vi "get_message.vi"(8 "error in (no error)":errorcluster, 11 "MoAgSy_Message.lvclass in":refnum<class "MoAgSy_Message.lvclass">) -> (0 "error out":errorcluster, 2 "Message":string, 3 "MoAgSy_Message.lvclass out":refnum<class "MoAgSy_Message.lvclass">)   [LabVIEW 2009, in "MoAgSy.lvlib" / "MoAgSy_Message.lvclass"]
uses:
  MoAgSy_Message.lvclass
  MoAgSy_Message.lvclass/MoAgSy_Message.ctl
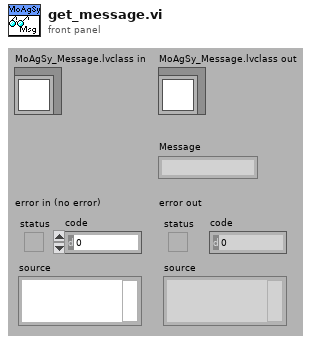
[diagram p1: front panel]
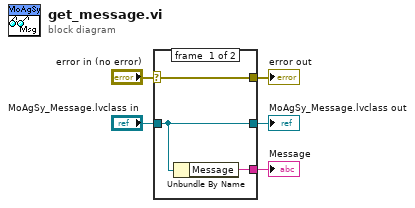
[diagram p0: block diagram]
diagram:
  n1 = case shown="No Error" "error in (no error)" {
    selector: "error in (no error)" -> [w8 w9]
    tunnel: [w8 w9] -> w4
    tunnel: [w7 w10] -> w2
    tunnel: "MoAgSy_Message.lvclass in" -> [w7 w10]
    tunnel: [w6 _] -> w1
    frame #0 {
      n2 = Unbundle By Name(w7) -> ("Message"=w6:string)
    }
    frame #1 {
    }
  }
  "error out" <- w4
  "MoAgSy_Message.lvclass out" <- w2
  "Message" <- w1
